vi "Test Epoch Conversion.vi"() -> ()   [LabVIEW 2018, in "InfluxDB Client.lvlib"]
uses:
  Controls/Precision.ctl
  InfluxDB Client.lvlib
panel:
  in  "Precision":T1
  out "Time Stamp (UTC)":timestamp format="%<%H:%M:%S%3u\n%Y/%m/%d>T"
  out "Time Stamp":timestamp format="%<%H:%M:%S%3u\n%Y/%m/%d>T"
  out "equal":bool
  in  "Unix epoch time":u64=1518555681
  out "Unix epoch time converted":u64
  # "13.2.2018, 22:06:20 local\n13.2.2018, 21:06:20 UTC"
  # "1518557595227349760"
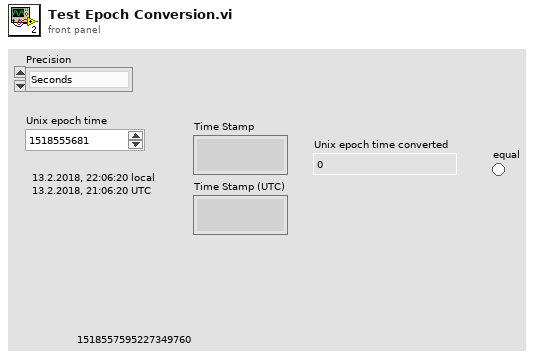
[diagram p1: front panel]
types:
  T1 = typedef "InfluxDB Client.lvlib/Precision.ctl" = enum16{"Seconds", "Milliseconds", "Nanoseconds"}
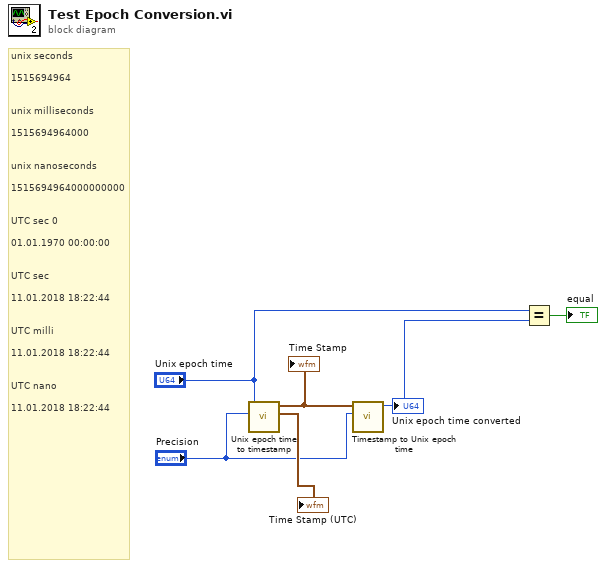
[diagram p0: block diagram]
diagram:
  # "unix seconds\n\n1515694964 \n\n\nunix milliseconds\n\n1515694964000 \n\n\nunix nanoseconds\n\n1515694964000000000 \n\n\nUTC sec 0\n\n01.01.1970 00:00:00 \n\n\nUTC sec\n\n11.01.2018 18:22:44 \n\n\nUTC milli\n\n11.01.2018 18:22:44 \n\n\nUTC nano\n\n11.01.2018 18:22:44"
  n1 = call "Unix epoch time to timestamp.vi"("Precision"="Precision", "Unix epoch time"="Unix epoch time") -> ("Time Stamp (UTC)"=→"Time Stamp (UTC)":timestamp, "Time Stamp"=w5:timestamp)  [unwired: 8 in]
  "Time Stamp" <- w5
  n2 = call "Timestamp to Unix epoch time.vi"("Precision (ns)"="Precision", "Timestamp"=w5) -> ("Unix epoch time"=w1:u64)  [unwired: 9 in]
  "Unix epoch time converted" <- w1
  n3 = Equal?(x="Unix epoch time", y=w1) -> (x = y?=→"equal":bool)
